vi "表格数据输入(数值)-8.6.vi"(6 "行数?":bool, 8 "行数":u32=1, 9 "列数":u32=1, 10 "数值数组":dbl[](array[numeric])=[0.0, 0.0, 0.0], 11 "表格引用":refnum<vi>) -> ()   [LabVIEW 2013]
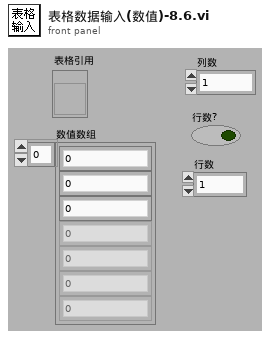
[diagram p1: front panel]
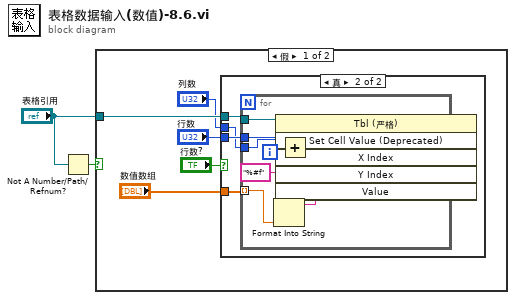
[diagram p0: block diagram]
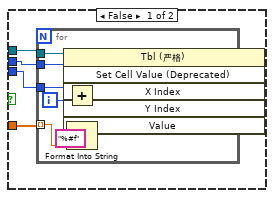
[diagram p2: hidden frame]
diagram:
  n1 = Not A Number/Path/Refnum?(number/path/refnum="表格引用") -> (NaN/Path/Refnum?=w2:bool)
  n2 = case shown="假" w2 {
    tunnel: "表格引用" -> [w6 _]
    frame False {
      n3 = case shown="真" "行数?" {
        tunnel: "数值数组" -> [w11 w23]
        tunnel: w6 -> [w10 w22]
        tunnel: "行数" -> [w9 w21]
        tunnel: "列数" -> [w8 w20]
        frame False {
          n4 = for {
            tunnel: w10 -> [w19]
            tunnel: w11 -> [w16] mode=indexing
            tunnel: w9 -> [w13]
            tunnel: w8 -> [w12]
            i -> [w18]
            n5 = Add(x=w13, y=w18) -> (x+y=w14:u32)
            n6 = Format Into String(format string="%#f" ("格式字符串"), w16) -> (resulting string=w15:string)  [unwired: 2 in, 1 out]
            n7 = invoke class="Tbl (严格)" method="Set Cell Value (Deprecated)"(reference=w19, "X Index"=w12, "Y Index"=w14, "Value"=w15) -> ()  [unwired: 2 in, 6 out]
          }
        }
        frame True {
          n8 = for {
            tunnel: w22 -> [w31]
            tunnel: w23 -> [w29] mode=indexing
            tunnel: w21 -> [w26]
            tunnel: w20 -> [w24]
            i -> [w30]
            n9 = Format Into String(format string="%#f" ("格式字符串"), w29) -> (resulting string=w28:string)  [unwired: 2 in, 1 out]
            n10 = Add(x=w24, y=w30) -> (x+y=w25:u32)
            n11 = invoke class="Tbl (严格)" method="Set Cell Value (Deprecated)"(reference=w31, "X Index"=w25, "Y Index"=w26, "Value"=w28) -> ()  [unwired: 2 in, 6 out]
          }
        }
      }
    }
    frame True {
    }
  }
